vi "appendix_getImageData.vi"(8 "TableData":T1[](array[typedef]), 9 "Pattern":string, 10 "filenames":string[](array[string]), 11 "path in":path) -> (3 "Data":T2[](array[typedef]))   [LabVIEW 2016]
uses:
  appendix_data.ctl
  WorReport_tableData.ctl
  WorReport_imageData.ctl
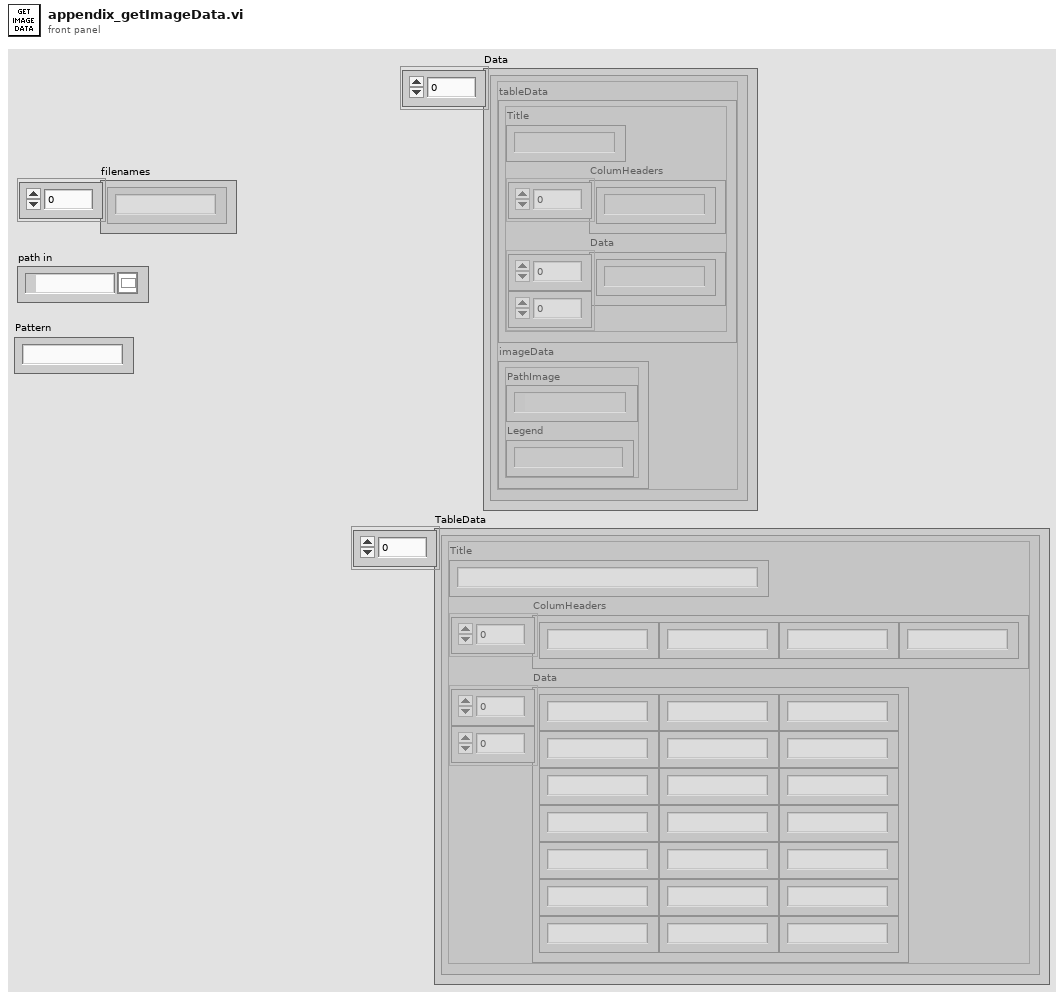
[diagram p1: front panel]
types:
  T1 = typedef "WorReport_tableData.ctl" = cluster{"Title":string, "ColumHeaders":string[], "Data":string[][]}
  T2 = typedef "appendix_data.ctl" = cluster{"tableData":T1, "imageData":T3}
  T3 = typedef "WorReport_imageData.ctl" = cluster{"PathImage":path, "Legend":string}
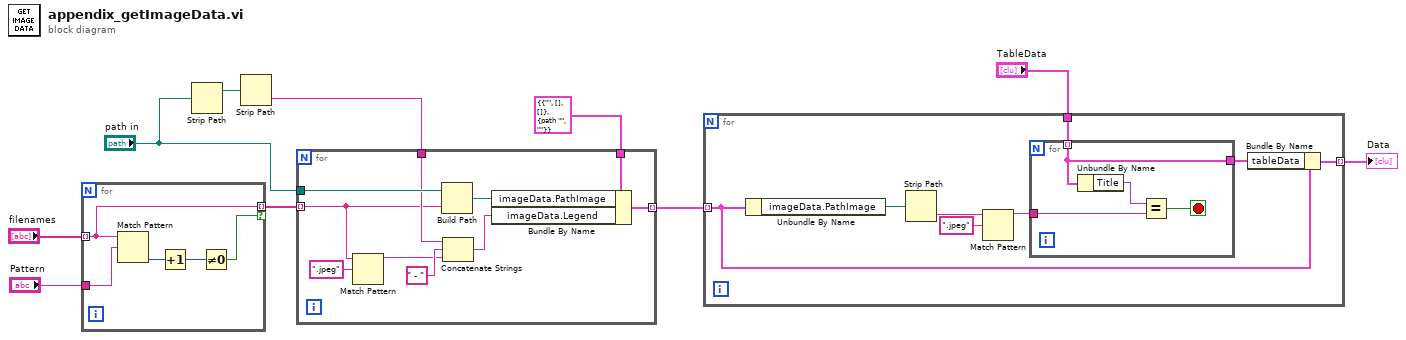
[diagram p0: block diagram]
diagram:
  n1 = for {
    tunnel: "filenames" -> [w11] mode=indexing
    tunnel: "Pattern" -> [w15]
    tunnel: [w11] -> w8 mode=indexing if=w12
    n2 = Match Pattern(string=w11, regular expression=w15) -> (offset past match=w14:i32)  [unwired: 1 in, 3 out]
    n3 = Increment(x=w14) -> (x+1=w13:i32)
    n4 = Not Equal To 0?(x=w13) -> (x != 0?=w12:bool)
  }
  n5 = Strip Path(path="path in") -> (stripped path=w9:path)  [unwired: 1 out]
  n6 = Strip Path(path=w9) -> (name=w5:string)  [unwired: 1 out]
  n7 = for {
    tunnel: w8 -> [w18] mode=indexing
    tunnel: "path in" -> [w25]
    tunnel: T2 {"tableData"={"Title"="", "ColumHeaders"=[], "Data"=[]}, "imageData"={"PathImage"=path "", "Legend"=""}} ("ImageData") -> [w24]
    tunnel: w5 -> [w22]
    tunnel: [w17] -> w4 mode=indexing
    n8 = Match Pattern(string=w18, regular expression=".jpeg") -> (before substring=w16:string)  [unwired: 1 in, 3 out]
    n9 = Build Path(base path=w25, name or relative path=w18) -> (appended path=w23:path)
    n10 = Concatenate Strings(w22, " - " ("string"), w16) -> (w20:string)
    n11 = Bundle By Name(cluster=w24, "imageData.PathImage"=w23, "imageData.Legend"=w20) -> (w17:T2)
  }
  n12 = for {
    tunnel: w4 -> [w28] mode=indexing
    tunnel: "TableData" -> [w30]
    tunnel: [w26] -> w2 mode=indexing
    n13 = Unbundle By Name(w28) -> ("imageData.PathImage"=w33:path)
    n14 = Strip Path(path=w33) -> (name=w32:string)  [unwired: 1 out]
    n15 = Match Pattern(string=w32, regular expression=".jpeg") -> (before substring=w29:string)  [unwired: 1 in, 3 out]
    n16 = for {
      tunnel: w30 -> [w34] mode=indexing
      tunnel: w29 -> [w36]
      tunnel: [w34] -> w27
      stop <- w35 stop-if-true
      n17 = Unbundle By Name(w34) -> ("Title"=w37:string)
      n18 = Equal?(x=w37, y=w36) -> (x = y?=w35:bool)
    }
    n19 = Bundle By Name(cluster=w28, "tableData"=w27) -> (w26:T2)
  }
  "Data" <- w2
